vi "TestLatchingBool_UserPressCaught.vi"(8 "error in (no error)":errorcluster, 11 "TestCase in":refnum<class "UITestAutoRegistration.lvclass">) -> (0 "error out":errorcluster, 3 "TestCase out":refnum<class "UITestAutoRegistration.lvclass">)   [LabVIEW 2017, in "UITestAutoRegistration.lvclass"]
uses:
  UITestAutoRegistration.lvclass
  C:/Program Files (x86)/National Instruments/LabVIEW 2017/vi.lib/addons/_JKI Toolkits/VI Tester/TestCase.llb/TestCase.lvclass
  <vilib>/addons/_JKI Toolkits/VI Tester/TestCase.llb/TestCase.lvclass
  Source/Framework/ActorEvents/AutoRegistration/AutoRegistration.lvclass
panel:
  in  "OK Button":bool
  # "Press latching button"
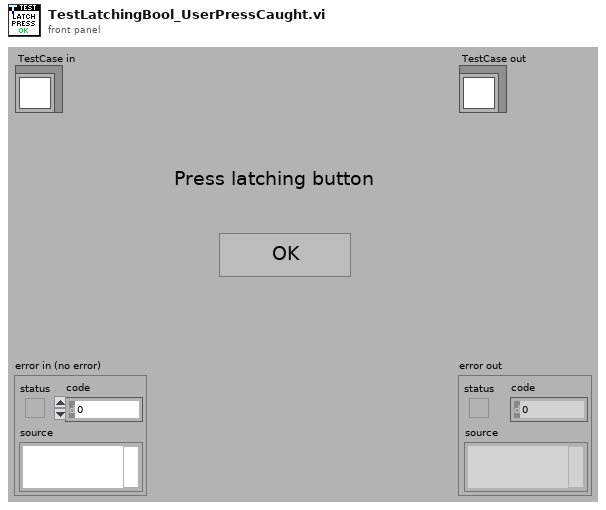
[diagram p1: front panel]
types:
  T1 = typedef "AutoRegistration.lvlib/AutoRegistration.lvclass/Auto-Event Registration Refnum.ctl" = refnum<event-registration>
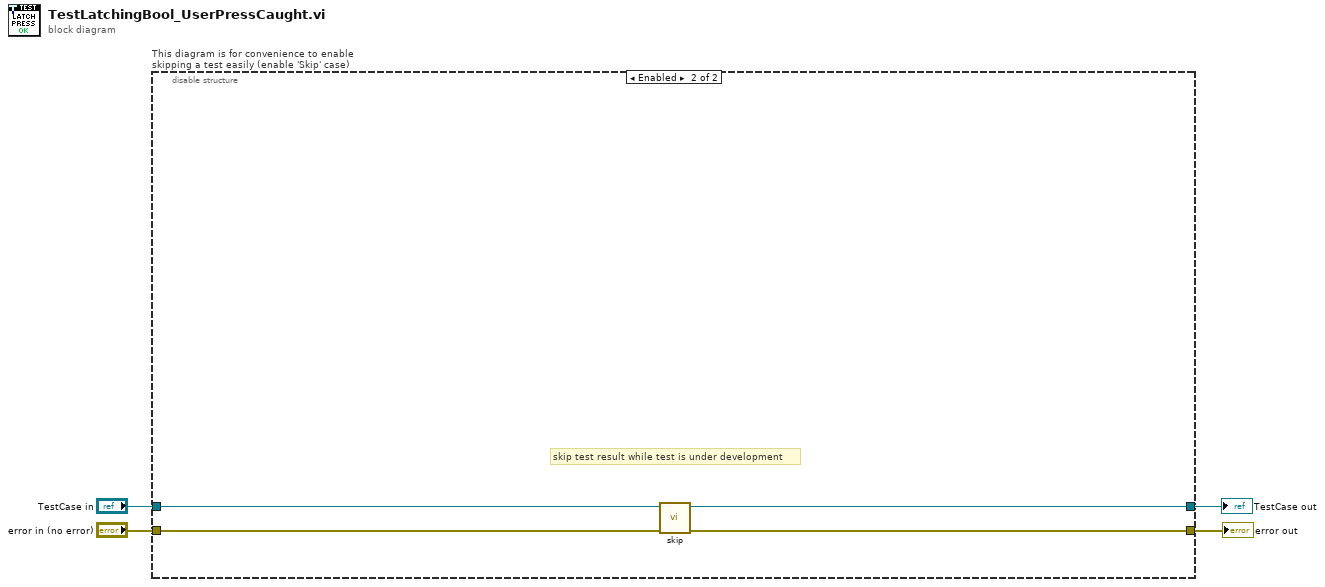
[diagram p0: block diagram]
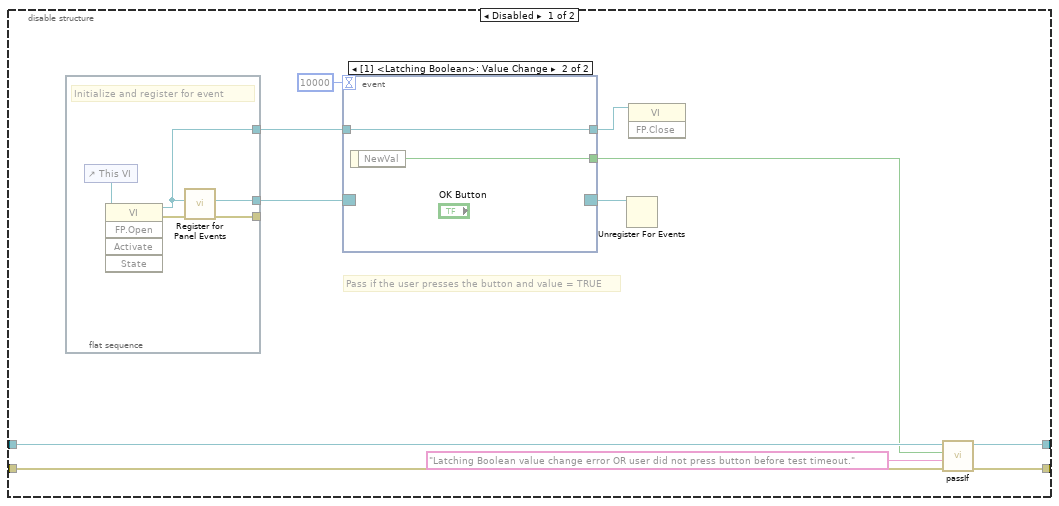
[diagram p2: hidden frame]
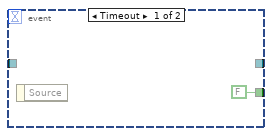
[diagram p3: hidden frame]
diagram:
  n1 = disable-structure "This diagram is for convenience to enable skipping a test easily (enable 'Skip' case)" shown="Enabled" {
    disable-tunnel: "TestCase in" -> [w15 w27]
    disable-tunnel: [w14 w25] -> w1
    disable-tunnel: [w13 w26] -> w3
    disable-tunnel: "error in (no error)" -> [w12 w24]
    frame Disabled {
      # "Pass if the user presses the button and value = TRUE"
      n2 = flat-sequence {
        tunnel: [w23] -> _
        tunnel: [w22] -> w11
        tunnel: [w19] -> w6
        frame #0 {
          # "Initialize and register for event"
          n3 = control-ref of="This VI"() -> (w21:refnum<vi>)
          n4 = invoke class="VI" method="FP.Open"(reference=w21) -> (reference out=w19:refnum<vi>, error out=w20:errorcluster)  [unwired: 4 in, 3 out]
          n5 = call "Register for Panel Events.vi"("error in (no error)"=w20, "VI Refnum (Calling VI)"=w19) -> ("error out"=w23:errorcluster, "Auto-Event Registration Refnum"=w22:T1)  [unwired: 6 in, 2 out]
        }
      }
      n6 = event shown="[1] <Latching Boolean>: Value Change" {
        selector: w11 -> [_ _]
        dyn-events: [_ _] -> w10
        timeout: 10000 -> [_ _]
        tunnel: [FALSE ("NewVal") w18] -> w8
        tunnel: w6 -> [_ w17]
        tunnel: [_ w17] -> w5
        event Timeout {
          n7 = event-data() -> ()  [unwired: 1 in, 1 out]
        }
        event Value Change {
          n8 = event-data() -> ("NewVal"=w18:bool)  [unwired: 1 in]
        }
      }
      n9 = Unregister For Events(event registration refnum=w10) -> ()  [unwired: 1 in, 1 out]
      n10 = invoke class="VI" method="FP.Close"(reference=w5) -> ()  [unwired: 2 in, 3 out]
      n11 = call-dynamic "passIf.vi"("error in (no error)"=w12, "message (\"\")"="Latching Boolean value change error OR user did not press button before test timeout." ("message (\"\")"), "pass"=w8, "TestCase in"=w15) -> ("error out"=w13:errorcluster, "TestCase out"=w14:refnum<class "UITestAutoRegistration.lvclass">)  [unwired: 6 in]
    }
    frame Enabled {
      # "skip test result while test is under development"
      n12 = call <vilib>:"skip.vi"("error in (no error)"=w24, "TestCase in"=w27) -> ("error out"=w26:errorcluster, "TestCase out"=w25:refnum<class "UITestAutoRegistration.lvclass">)  [unwired: 8 in]
    }
  }
  "error out" <- w3
  "TestCase out" <- w1
